vi "Create.vi"(8 "error in (no error)":errorcluster, 10 "Messages":set{string}(c389)) -> (0 "error out":errorcluster, 3 "Filter by Process out":refnum<class "Filter by Message.lvclass">)   [LabVIEW 2020, in "Filter by Message.lvclass"]
uses:
  Filter by Message.lvclass
  Filter by Message.lvclass/Filter by Message.ctl
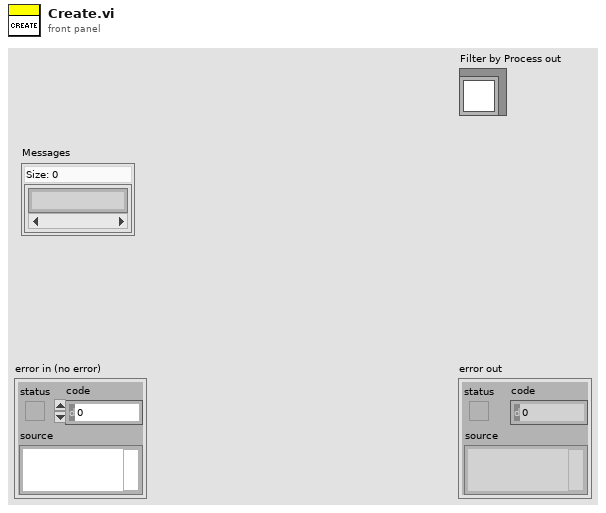
[diagram p1: front panel]
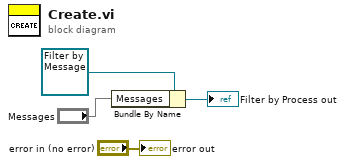
[diagram p0: block diagram]
diagram:
  n1 = Bundle By Name(cluster=refnum<class "Filter by Message.lvclass"> refnum ("Filter by Process out"), "Messages"="Messages") -> (→"Filter by Process out":refnum<class "Filter by Message.lvclass">)
  "error out" <- "error in (no error)"
